vi "Convert TableItems to StringType ColumeNames.vi"(8 "error in (no error)":errorcluster, 11 "ScriptDatabase in":refnum<class "ScriptDatabase.lvclass">) -> (0 "error out":errorcluster, 3 "ScriptDatabase out":refnum<class "ScriptDatabase.lvclass">)   [LabVIEW 2015, in "ScriptDatabase.lvclass"]
uses:
  ScriptDatabase.lvclass
  ScriptDatabase.lvclass/ScriptDatabase.ctl
  <vilib>/addons/database/Auxilliary.llb/DB Tools DataTypes.ctl
  <vilib>/addons/database/NI_Database_API.lvlib
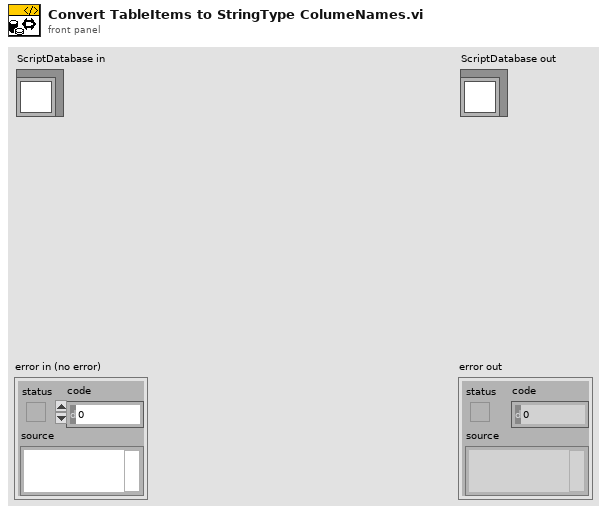
[diagram p1: front panel]
types:
  T1 = typedef "NI_Database_API.lvlib/DB Tools DataTypes.ctl" = enum16{"String", "Long (I32)", "Single (SGL)", "Double (DBL)", "Date/Time", "Binary"}
  T2 = typedef "NI_Database_API.lvlib/DB Tools Column Info.ctl" = cluster{"column name":string, "data type":T1, "size":i32, "allow null?":bool}
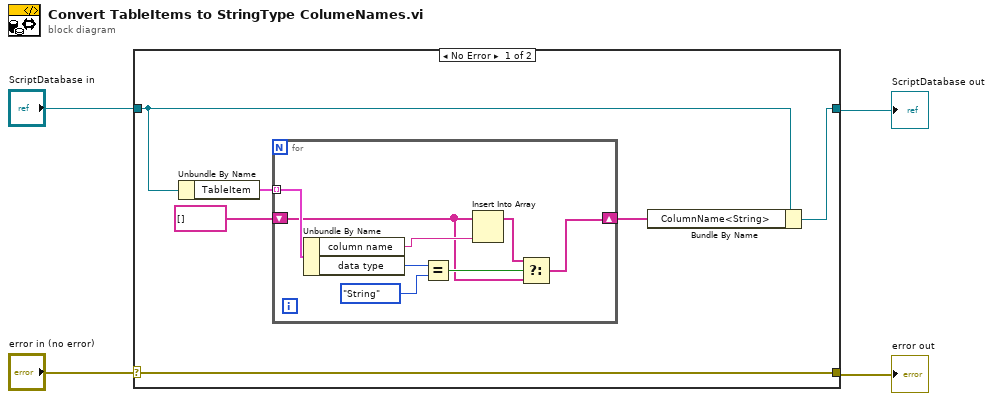
[diagram p0: block diagram]
diagram:
  n1 = case shown="No Error" "error in (no error)" {
    selector: "error in (no error)" -> [w10 w20]
    tunnel: [w10 w20] -> w3
    tunnel: [w5 w19] -> w1
    tunnel: "ScriptDatabase in" -> [w7 w19]
    frame No Error {
      n2 = Unbundle By Name(w7) -> ("TableItem"=w9:T2[])
      n3 = for {
        tunnel: w9 -> [w18] mode=indexing
        shift-right: [w11] -> w6
        shift-left: string[] [] ("column name") -> [w12]
        n4 = Unbundle By Name(w18) -> ("column name"=w16:string, "data type"=w17:T1)
        n5 = Equal?(x=w17, y=DB_Tools_DataTypes."String") -> (x = y?=w14:bool)
        n6 = Insert Into Array(array=w12, new element=w16) -> (w13:string[])  [unwired: 1 in]
        n7 = Select(t=w13, s=w14, f=w12) -> (s? t:f=w11:string[])
      }
      n8 = Bundle By Name(cluster=w7, "ColumnName<String>"=w6) -> (w5:refnum<class "ScriptDatabase.lvclass">)
    }
    frame Error {
    }
  }
  "error out" <- w3
  "ScriptDatabase out" <- w1
